vi "get_counter_settings.vi"(8 "error in (no error)":errorcluster, 11 "TrajectoryDL090201FrameScan in":refnum<class "TrajectoryDL090201FrameScan.lvclass">) -> (0 "error out":errorcluster, 2 "counter settings":T1[](array[typedef]), 3 "TrajectoryDL090201FrameScan out":refnum<class "TrajectoryDL090201FrameScan.lvclass">)   [LabVIEW 2010, in "TrajectoryDL090201FrameScan.lvclass"]
uses:
  TrajectoryDL090201FrameScan.lvclass
  common/clusters/counter_settings_cluster.ctl
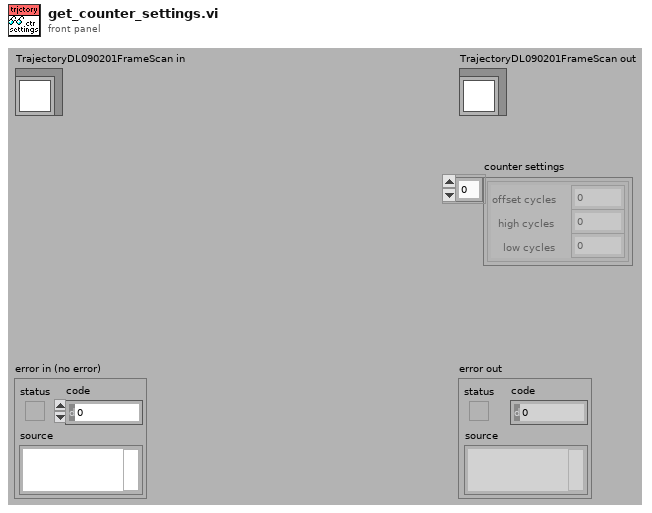
[diagram p1: front panel]
types:
  T1 = typedef "counter_settings_cluster.ctl" = cluster{"offset cycles":i32, "high cycles":i32, "low cycles":i32}
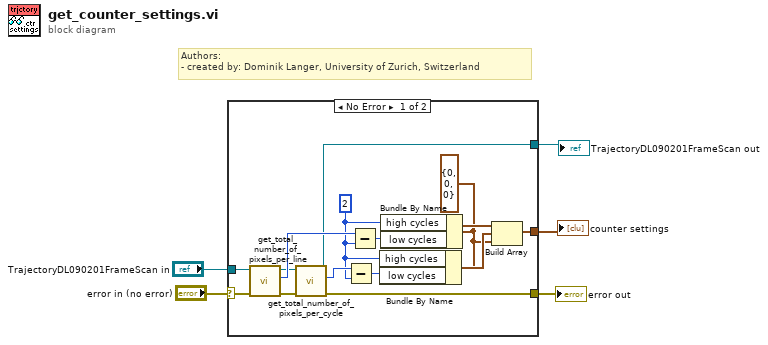
[diagram p0: block diagram]
diagram:
  # "Authors: \n- created by: Dominik Langer, University of Zurich, Switzerland"
  n1 = case shown="No Error" "error in (no error)" {
    selector: "error in (no error)" -> [w20 w22]
    tunnel: "TrajectoryDL090201FrameScan in" -> [w19 w21]
    tunnel: [w13 w22] -> w2
    tunnel: [w11 w21] -> w3
    tunnel: [w15 _] -> w1
    frame No Error {
      w6 = 2 ("high cycles")
      w9 = T1 {"offset cycles"=0, "high cycles"=0, "low cycles"=0} ("counter")
      n2 = call-dynamic "get_total_number_of_pixels_per_line.vi"("error in (no error)"=w20, "DL090201FrameScanTrajectory in"=w19) -> ("error out"=w14:errorcluster, "total number of pixels per line"=w18:i32, "DL090201FrameScanTrajectory out"=w12:refnum<class "TrajectoryDL090201FrameScan.lvclass">)  [unwired: 7 in]
      n3 = call-dynamic "get_total_number_of_pixels_per_cycle.vi"("error in (no error)"=w14, "TrajectoryDL090201FrameScan in"=w12) -> ("error out"=w13:errorcluster, "total number of pixels per cycle"=w7:i32, "TrajectoryDL090201FrameScan out"=w11:refnum<class "TrajectoryDL090201FrameScan.lvclass">)  [unwired: 7 in]
      n4 = Subtract(x=w7, y=w6) -> (x-y=w8:i32)
      n5 = Subtract(x=w18, y=w6) -> (x-y=w17:i32)
      n6 = Bundle By Name(cluster=w9, "high cycles"=w6, "low cycles"=w8) -> (w10:T1)
      n7 = Bundle By Name(cluster=w9, "high cycles"=w6, "low cycles"=w17) -> (w16:T1)
      n8 = Build Array(w16, w10, w9) -> (w15:T1[])
    }
    frame Error {
    }
  }
  "error out" <- w2
  "TrajectoryDL090201FrameScan out" <- w3
  "counter settings" <- w1
